vi "refMgr_Example3.2.vi"() -> ()   [LabVIEW 2017]
uses:
  RefManager/TagDB RefManager.lvlib
  <userlib>/_NEVSTOP/TagDB/TagDB.lvlib
panel:
  in  "aaa":string="aaaa"
  in  "toggle":bool
  in  "stop":bool
  in  "Boolean 0":bool
  in  "StateValue":i32
  in  "Boolean 5":bool
  in  "Boolean 4":bool
  in  "Boolean 3":bool
  in  "Boolean 2":bool
  in  "Boolean 1":bool
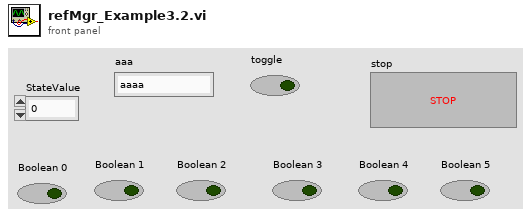
[diagram p1: front panel]
types:
  T1 = typedef "TagDB.lvlib/TagDB.ctl" = refnum<k1>
  T2 = typedef "TagDB RefManager.lvlib/RefMgr-Logic-State.ctl" = cluster{"StateName":string, "StateValue":i32, "Type":T3, "Calcs":cluster{"Tag":string, "Exp":string}[]}
  T3 = typedef "TagDB RefManager.lvlib/RefMgr-StateChangeType.ctl" = enum16{"0 - 进入", "1 - 等于", "2 - 退出"}
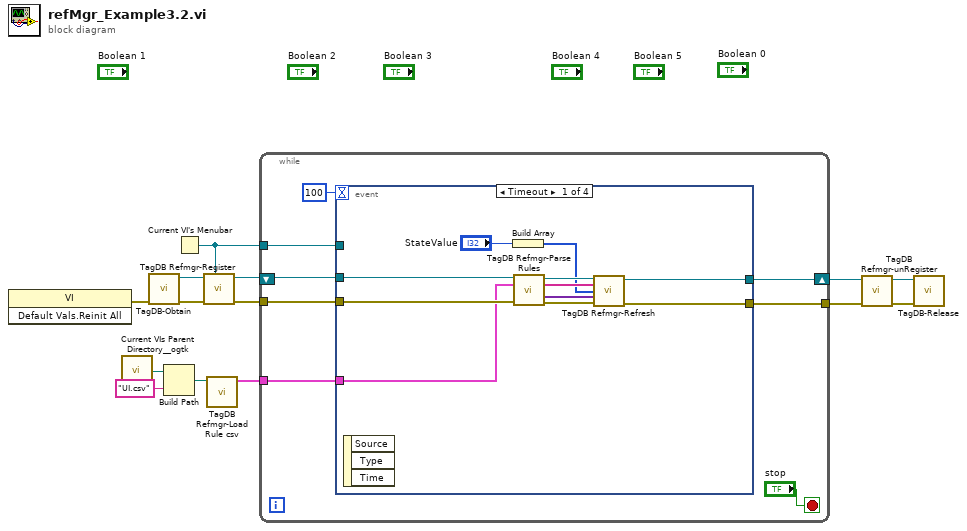
[diagram p0: block diagram]
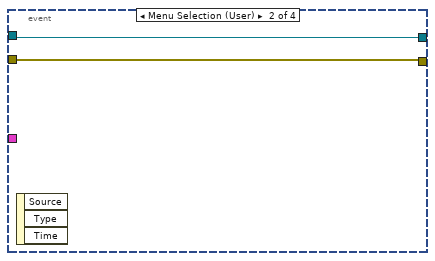
[diagram p2: hidden frame]
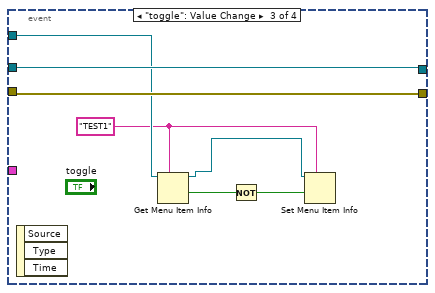
[diagram p3: hidden frame]
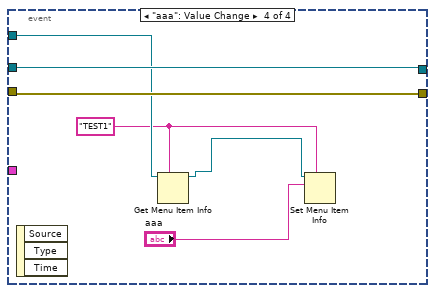
[diagram p4: hidden frame]
diagram:
  n1 = invoke class="VI" method="Default Vals.Reinit All"() -> (error out=w6:errorcluster)  [unwired: 3 in, 2 out]
  n2 = call <userlib>:"Current VIs Parent Directory__ogtk.vi"() -> ("Parent Directory (+ Relative)"=w3:path)  [unwired: 5 in]
  n3 = call <userlib>:"TagDB-Obtain.vi"("error in (no error)"=w6) -> ("error out"=w13:errorcluster, "TagDB"=w14:T1)  [unwired: 4 in, 1 out]
  n4 = Build Path(base path=w3, name or relative path="UI.csv") -> (appended path=w2:path)
  n5 = Current VI's Menubar() -> (w5:refnum<k9>)
  n6 = call "TagDB Refmgr-Register.vi"("menu reference"=w5, "error in (no error)"=w13, "TagDB in"=w14) -> ("error out"=w11:errorcluster, "TagDB out"=w12:T1)  [unwired: 6 in, 1 out]
  n7 = call "TagDB Refmgr-Load Rule csv.vi"("Path"=w2) -> ("Array 2"=w4:T2[])  [unwired: 9 in, 1 out]
  n8 = while {
    tunnel: w11 -> [w21]
    tunnel: w4 -> [w20]
    tunnel: [w17] -> w9
    shift-right: [w18] -> w10
    shift-left: w12 -> [w22]
    tunnel: w5 -> [w15]
    stop <- "stop" stop-if-true
    n9 = event shown="[0] Timeout" {
      selector: _ -> [_ _ _ _]
      dyn-events: _ -> [_ _ _ _]
      timeout: 100 -> [_ _ _ _]
      tunnel: w22 -> [w33 w35 w42 w48]
      tunnel: w21 -> [w32 w34 w41 w47]
      tunnel: w20 -> [w31 _ _ _]
      tunnel: [w24 w35 w42 w48] -> w18
      tunnel: [w23 w34 w41 w47] -> w17
      tunnel: w15 -> [_ _ w39 w45]
      event Timeout {
        n10 = event-data() -> ()  [unwired: 1 in, 3 out]
        n11 = Build Array("StateValue") -> (w25:i32[])
        n12 = call "TagDB Refmgr-Parse Rules.vi"("DB Ref"=w33, "Rules"=w31, "error in (no error)"=w32) -> ("DB Ref (dup)"=w30:T1, "StateNames"=w28:string[], "RulesMap"=w27:variant[], "error out"=w29:errorcluster)  [unwired: 9 in]
        n13 = call "TagDB Refmgr-Refresh.vi"("DB Ref"=w30, "StateName"=w28, "State"=w25, "RulesMap"=w27, "error in (no error)"=w29) -> ("DB Ref (dup)"=w24:T1, "error out"=w23:errorcluster)  [unwired: 9 in]
      }
      event Menu Selection (User) {
        n14 = event-data() -> ()  [unwired: 1 in, 3 out]
      }
      event "toggle": Value Change {
        w38 = "TEST1" ("item name")
        n15 = event-data() -> ()  [unwired: 1 in, 3 out]
        n16 = Get Menu Item Info(7:w38, 11:w39) -> (1:w37:bool, 3:w40:refnum<k9>)  [unwired: 1 in, 5 out]
        n17 = Not(x=w37) -> (.not. x?=w36:bool)
        n18 = Set Menu Item Info(7:w38, 9:w36, 11:w40) -> ()  [unwired: 4 in, 2 out]
      }
      event "aaa": Value Change {
        w44 = "TEST1" ("item name")
        n19 = event-data() -> ()  [unwired: 1 in, 3 out]
        n20 = Get Menu Item Info(7:w44, 11:w45) -> (3:w46:refnum<k9>)  [unwired: 1 in, 6 out]
        n21 = Set Menu Item Info(7:w44, 10:"aaa", 11:w46) -> ()  [unwired: 4 in, 2 out]
      }
    }
  }
  n22 = call "TagDB Refmgr-unRegister.vi"("error in (no error)"=w9, "TagDB in"=w10) -> ("error out"=w8:errorcluster, "TagDB out"=w7:T1)  [unwired: 8 in]
  n23 = call <userlib>:"TagDB-Release.vi"("error in (no error)"=w8, "TagDB"=w7) -> ()  [unwired: 9 in, 1 out]
